vi "Disconnect.vi"(8 "error in (no error)":errorcluster, 11 "UR5 Robot in":refnum<class "UR5 Robot.lvclass">) -> (0 "error out":errorcluster, 3 "UR5 Robot out":refnum<class "UR5 Robot.lvclass">)   [LabVIEW 2018, in "UR5 Robot.lvlib" / "UR5 Robot.lvclass"]
uses:
  UR5 Robot.lvclass
  UR5 Robot.lvclass/UR5 Robot.ctl
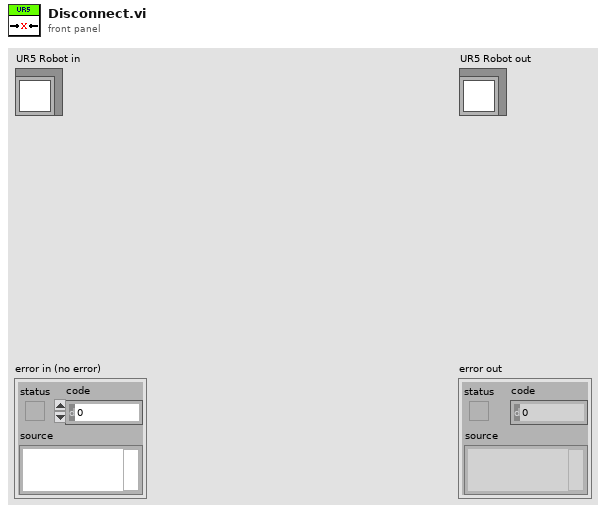
[diagram p1: front panel]
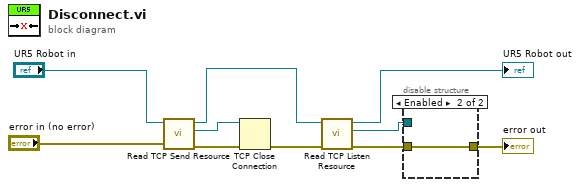
[diagram p0: block diagram]
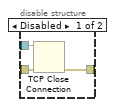
[diagram p2: hidden frame]
diagram:
  n1 = call "Read TCP Send Resource.vi"("error in (no error)"="error in (no error)", "UR5 Robot in"="UR5 Robot in") -> ("error out"=w8:errorcluster, "TCP Send Resource"=w3:refnum<k5>, "UR5 Robot out"=w5:refnum<class "UR5 Robot.lvclass">)  [unwired: 7 in]
  n2 = TCP Close Connection(connection ID=w3, error in (no error)=w8) -> (error out=w7:errorcluster)  [unwired: 1 in, 1 out]
  n3 = call "Read TCP Listen Resource.vi"("error in (no error)"=w7, "UR5 Robot in"=w5) -> ("error out"=w6:errorcluster, "TCP Listen Resource"=w2:refnum<k5>, "UR5 Robot out"=→"UR5 Robot out":refnum<class "UR5 Robot.lvclass">)  [unwired: 7 in]
  n4 = disable-structure shown="Enabled" {
    disable-tunnel: w6 -> [w13 w14]
    disable-tunnel: w2 -> [w12 _]
    disable-tunnel: [w11 w14] -> w1
    frame Disabled {
      n5 = TCP Close Connection(connection ID=w12, error in (no error)=w13) -> (error out=w11:errorcluster)  [unwired: 1 in, 1 out]
    }
    frame Enabled {
    }
  }
  "error out" <- w1
